vi "Write send to address.vi"(8 "error in (no error)":errorcluster, 10 "send to address":string="localhost", 11 "TEC configuration in":refnum<class "TEC configuration.lvclass">) -> (0 "error out":errorcluster, 3 "TEC configuration out":refnum<class "TEC configuration.lvclass">)   [LabVIEW 2013, in "TEC configuration.lvclass"]
uses:
  TEC configuration.lvclass
  TEC configuration.lvclass/TEC configuration.ctl
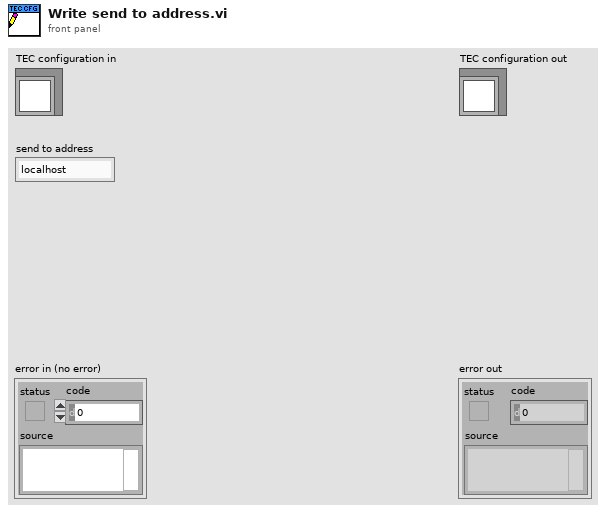
[diagram p1: front panel]
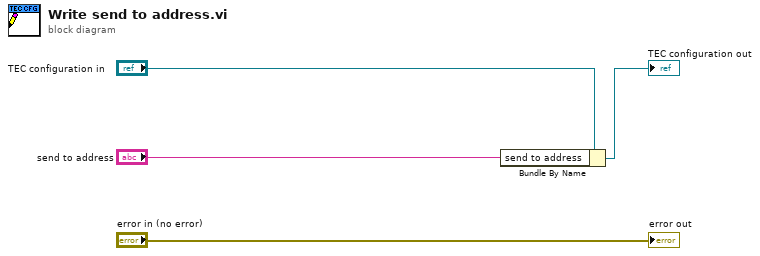
[diagram p0: block diagram]
diagram:
  n1 = Bundle By Name(cluster="TEC configuration in", "send to address"="send to address") -> (→"TEC configuration out":refnum<class "TEC configuration.lvclass">)
  "error out" <- "error in (no error)"
